vi "TestGridViewDotNET.vi"() -> ()   [LabVIEW 2013]
uses:
  Shared/LabVIEWdotNetDataGrid-master/source/GridColumn/ColumnDefinition.ctl
  Shared/LabVIEWdotNetDataGrid-master/source/GridColumn/ColumnType.ctl
  System.Windows.Forms
  Shared/LabVIEWdotNetDataGrid-master/source/DataGridView/DataGridView.lvclass
  Shared/LabVIEWdotNetDataGrid-master/source/Events/Abstract EVENT/Abstract EVENT.lvclass
  Shared/LabVIEWdotNetDataGrid-master/source/DataTable/DataTable.lvclass
  Shared/LabVIEWdotNetDataGrid-master/source/DataGridView/DataGridView.lvclass/DataGridView.ctl
  Shared/LabVIEWdotNetDataGrid-master/source/DataGridView/Properties/Read registeredEvents.vi
  Shared/LabVIEWdotNetDataGrid-master/source/DataTable/Add Rows (String).vi
  Shared/LabVIEWdotNetDataGrid-master/source/Events/CellValueChanged/CellValueChanged.lvclass
  Shared/LabVIEWdotNetDataGrid-master/source/Events/KeyDown/KeyDown.lvclass
  Shared/LabVIEWdotNetDataGrid-master/source/Events/CellClick/CellClick.lvclass
  Shared/LabVIEWdotNetDataGrid-master/source/GridColumn/GridColumn.lvclass
panel:
  in  "index":i32
  out "Events":string
  out "error out":errorcluster
  out "registeredEvents":refnum<event-registration>
  out "DataGrid out":refnum<class "DataGridView.lvclass">
  in  "error in":errorcluster
  in  "DataGridView":refnum<k24>(container)
  in  "ColumnSetup":T1[](array[typedef])=[{"name"="DeviceTypes", "caption"="DeviceTypes", "datatype"=enum."combo", "Params"="", "AutoSizeMode"=16, "FillWeight"=100.0, "MinWidth"=50, "tooltip"="DeviceTypes"}, {"name"="Devices", "caption"="Devices", "datatype"=enum."combo", "Params"="", "AutoSizeMode"=1, "FillWeight"=100.0, "MinWidth"=50, "tooltip"="Devices"}, {"name"="Variables", "caption"="Variables", "datatype"=enum."combo", "Params"="", "AutoSizeMode"=1, "FillWeight"=100.0, "MinWidth"=50, "tooltip"="Variables"}] {"MinWidth" min=2 step=1; "AutoSizeMode" items=["None"=1, "ColumnHeader"=2, "AllCellsExceptHeader"=4, "AllCells"=6, "DisplayedCellsExceptHeader"=8, "DisplayedCells"=10, "Fill"=16]; "FillWeight" min=1 max=100}
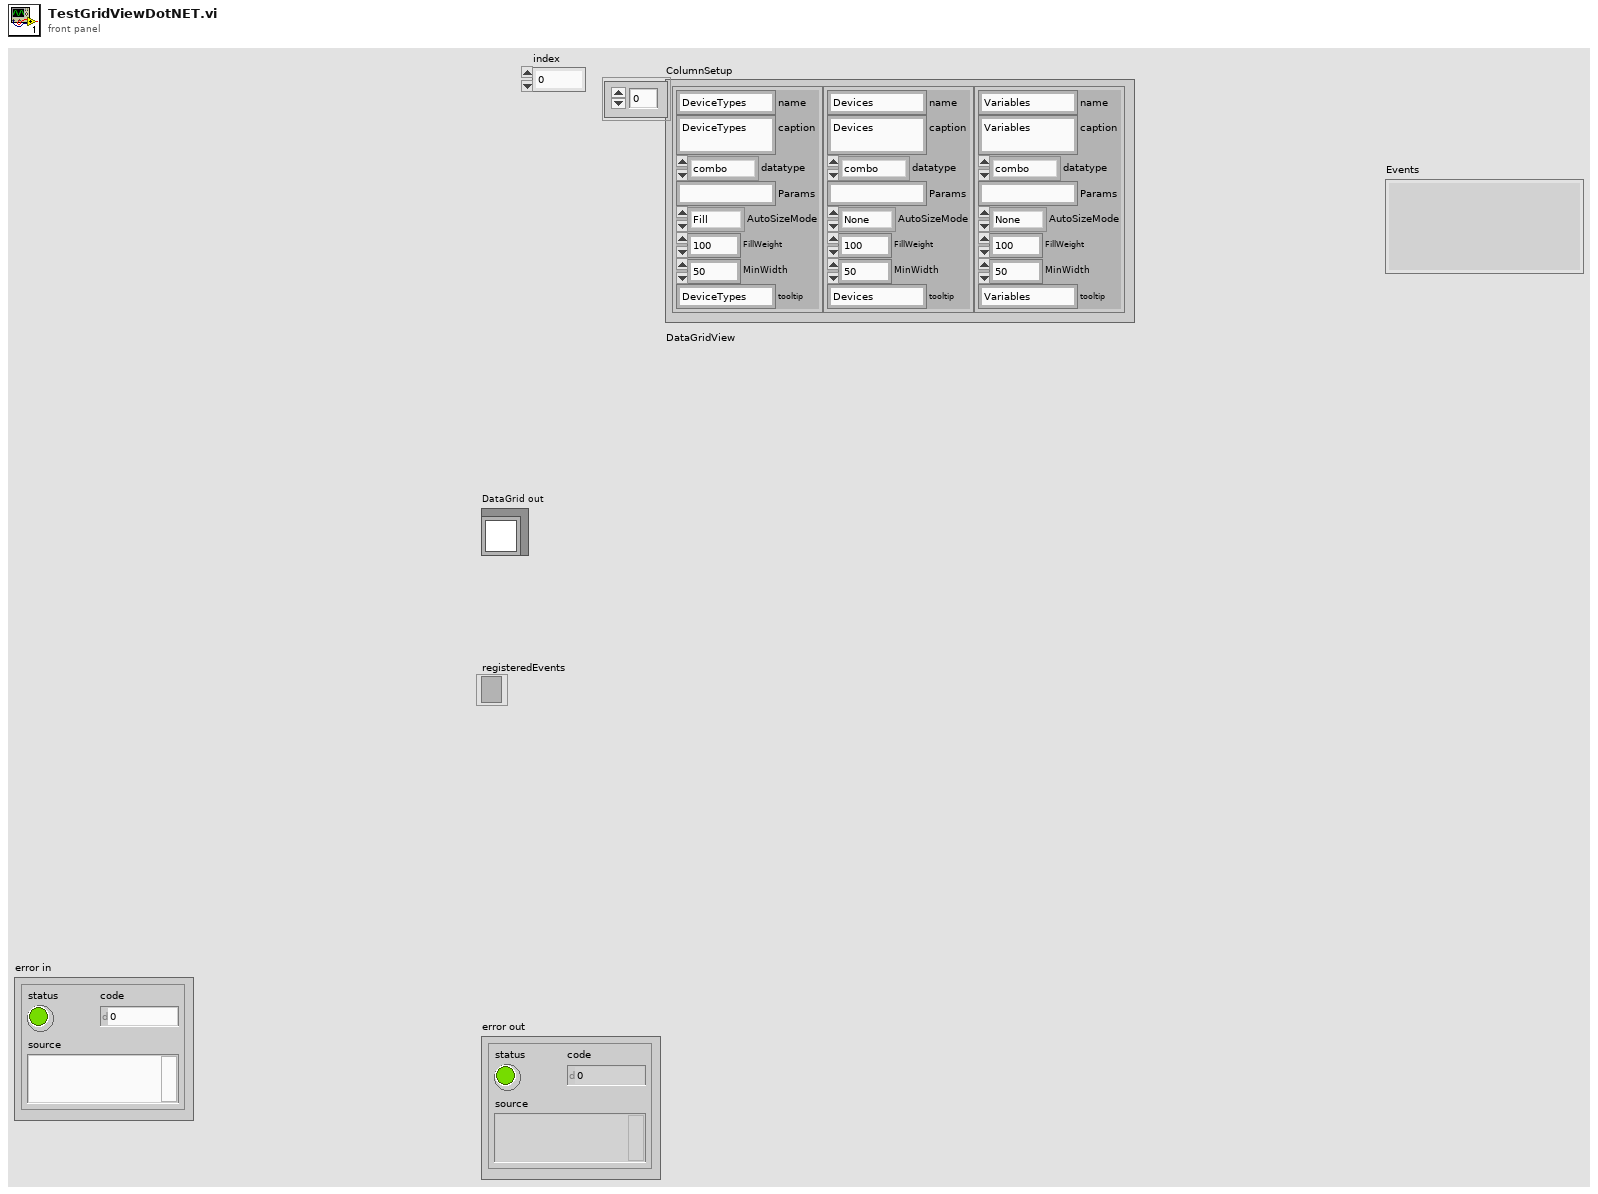
[diagram p1: front panel]
types:
  T1 = typedef "DataGrid.lvlib/GridColumn.lvclass/ColumnDefinition.ctl" = cluster{"name":string, "caption":string, "datatype":T2, "Params":string, "AutoSizeMode":i32, "FillWeight":sgl, "MinWidth":u32, "tooltip":string}
  T2 = typedef "DataGrid.lvlib/GridColumn.lvclass/ColumnType.ctl" = enum16{"string", "image", "check", "numeric", "timestamp", "button", "combo", "link"}
  T3 = cluster{"Alt":bool, "Control":bool, "KeyCode":i32, "KeyData":i32, "KeyValue":i32, "Modifiers":i32, "Shift":bool}
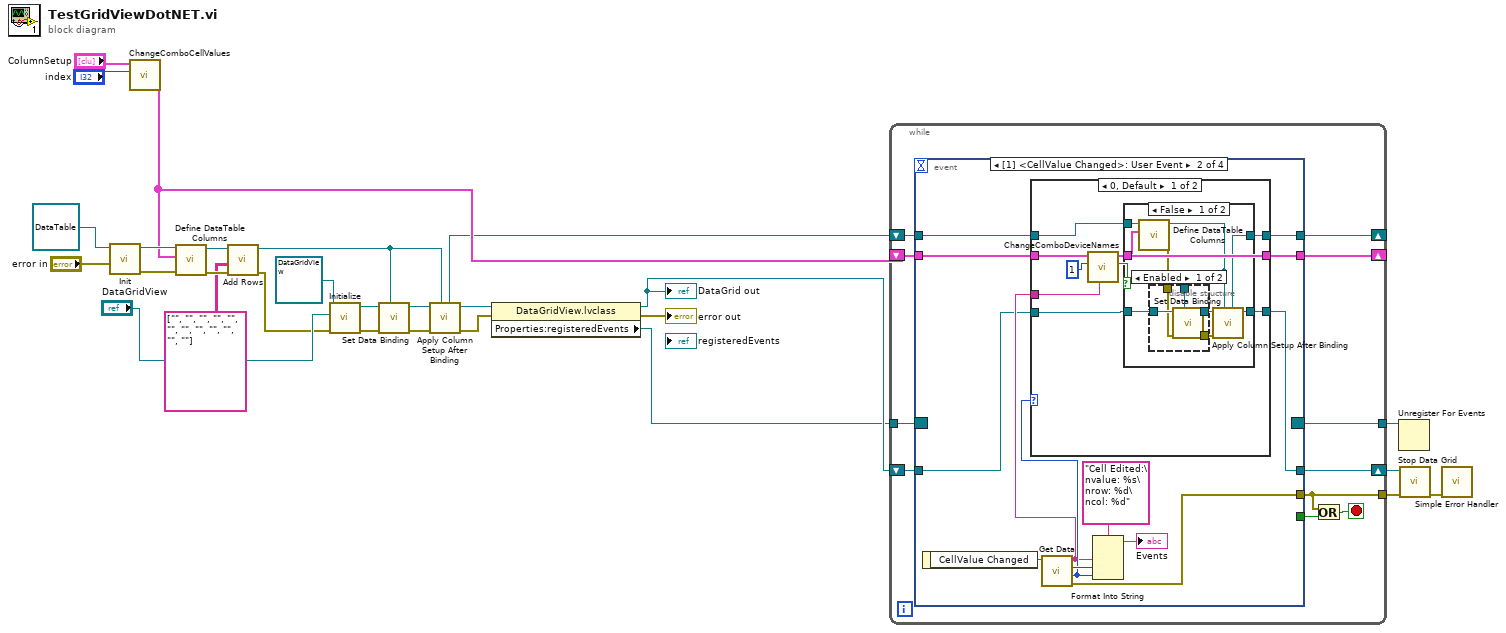
[diagram p0: block diagram]
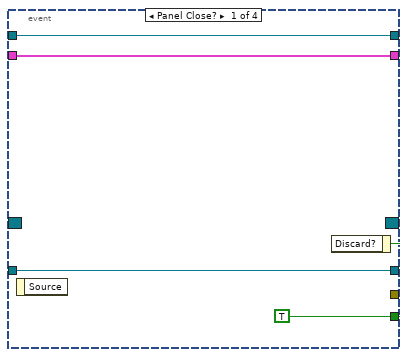
[diagram p2: hidden frame]
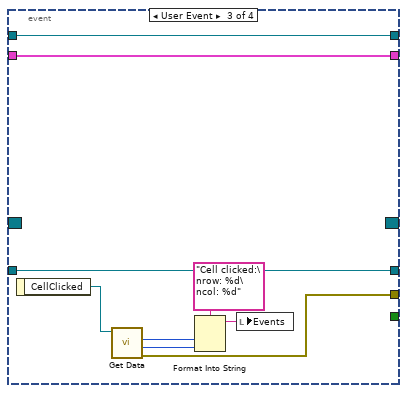
[diagram p6: hidden frame]
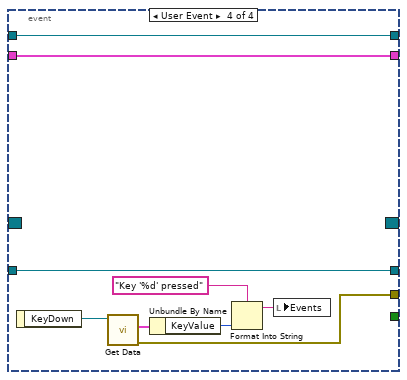
[diagram p7: hidden frame]
diagram:
  n1 = call "Init.vi"("error in (no error)"="error in", "DataTable in"=refnum<class "DataTable.lvclass"> refnum) -> ("error out"=w24:errorcluster, "DataTable out"=w25:refnum<class "DataTable.lvclass">)  [unwired: 8 in]
  n2 = call "ChangeComboCellValues.vi"("index"="index", "ColumnSetup in"="ColumnSetup") -> ("ColumnSetup out"=w5:T1[])  [unwired: 9 in]
  n3 = call "Define DataTable Columns.vi"("error in (no error)"=w24, "ColumnSetup"=w5, "DataTable In"=w25) -> ("error out"=w9:errorcluster, "DataTable Out"=w7:refnum<class "DataTable.lvclass">)  [unwired: 7 in]
  n4 = call-poly "Add Rows.vi"("error in (no error)"=w9, "String Data"=string[][] [["", "", ""], ["", "", ""], ["", "", ""], ["", "", ""]], "DataTable in"=w7) -> ("error out"=w8:errorcluster, "DataTable out"=w3:refnum<class "DataTable.lvclass">)  [unwired: 7 in]
  n5 = call "Initialize.vi"("error in"=w8, "DataGridView"="DataGridView", "DataGrid in"=refnum<class "DataGridView.lvclass"> refnum) -> ("error out"=w18:errorcluster, "DataGrid out"=w17:refnum<class "DataGridView.lvclass">)  [unwired: 7 in]
  n6 = call "Set Data Binding.vi"("DataTable Source"=w3, "error in (no error)"=w18, "DataGridView in"=w17) -> ("error out"=w21:errorcluster, "DataGridView out"=w23:refnum<class "DataGridView.lvclass">)  [unwired: 7 in]
  n7 = call "Apply Column Setup After Binding.vi"("DataTable"=w3, "error in (no error)"=w21, "DataGridView in"=w23) -> ("error out"=w19:errorcluster, "DataGridView out"=w22:refnum<class "DataGridView.lvclass">, "DataTable out"=w2:refnum<class "DataTable.lvclass">)  [unwired: 6 in]
  n8 = property class="DataGridView.lvclass"(reference=w22, error in=w19) -> (reference out=w10:refnum<class "DataGridView.lvclass">, error out=→"error out":errorcluster, "Properties:registeredEvents"=w1:refnum<event-registration>)
  "DataGrid out" <- w10
  n9 = while {
    tunnel: w1 -> [w39]
    shift-right: [w37] -> w12
    shift-left: w10 -> [w38]
    tunnel: [w36] -> w11
    tunnel: [w34] -> w13
    shift-right: [w31] -> _
    shift-left: w5 -> [w32]
    shift-right: [w29] -> _
    shift-left: w2 -> [w30]
    stop <- w33 stop-if-true
    n10 = event shown="[1] <CellValue Changed>: User Event" {
      selector: w39 -> [_ _ _ _]
      dyn-events: [_ _ _ _] -> w36
      timeout: _ -> [_ _ _ _]
      tunnel: [w43 _ _ _] -> w35
      tunnel: w38 -> [w42 w45 w94 w104]
      tunnel: [w42 w44 w94 w104] -> w37
      tunnel: [_ w52 w91 w98] -> w34
      tunnel: w32 -> [w41 w51 w88 w97]
      tunnel: [w41 w48 w88 w97] -> w31
      tunnel: w30 -> [w40 w47 w87 w96]
      tunnel: [w40 w46 w87 w96] -> w29
      event Panel Close? {
        w43 = TRUE ("Discard?")
        n11 = event-data() -> ()  [unwired: 1 in, 1 out]
        n12 = event-data("Discard?"=w43) -> ()  [unwired: 1 in, 1 out]
      }
      event User Event {
        n13 = event-data() -> ("CellValue Changed"=w54:refnum<class "Abstract EVENT.lvclass">)  [unwired: 1 in]
        n14 = call "Get Data.vi"("DataGrid.lvlib:Abstract EVENT.lvclass"=w54) -> ("error out"=w52:errorcluster, "column"=w50:i32, "row"=w53:i32, "cell value"=w49:string)  [unwired: 7 in]
        n15 = case shown="0, Default" w50 {
          tunnel: w51 -> [w65 w86]
          tunnel: w49 -> [w63 _]
          tunnel: [w58 w86] -> w48
          tunnel: w47 -> [w60 w85]
          tunnel: [w59 w85] -> w46
          tunnel: w45 -> [w61 w84]
          tunnel: [w62 w84] -> w44
          frame 0, Default {
            n16 = call "ChangeComboDeviceNames.vi"("DeviceTypeName"=w63, "index"=1, "ColumnSetup in"=w65) -> ("empty?"=w57:bool, "ColumnSetup out"=w58:T1[])  [unwired: 7 in]
            n17 = case shown="False" w57 {
              tunnel: [w74 w82] -> w62
              tunnel: w61 -> [w72 w82]
              tunnel: w60 -> [w70 w83]
              tunnel: [w66 w83] -> w59
              tunnel: w58 -> [w67 _]
              frame False {
                n18 = call "Define DataTable Columns.vi"("ColumnSetup"=w67, "DataTable In"=w70) -> ("error out"=w68:errorcluster, "DataTable Out"=w69:refnum<class "DataTable.lvclass">)  [unwired: 8 in]
                n19 = disable-structure shown="Enabled" {
                  disable-tunnel: [w79 w80] -> w73
                  disable-tunnel: w72 -> [w78 w81]
                  disable-tunnel: [w77 w81] -> w71
                  disable-tunnel: w69 -> [w76 _]
                  disable-tunnel: w68 -> [w75 w80]
                  frame Enabled {
                    n20 = call "Set Data Binding.vi"("DataTable Source"=w76, "error in (no error)"=w75, "DataGridView in"=w78) -> ("error out"=w79:errorcluster, "DataGridView out"=w77:refnum<class "DataGridView.lvclass">)  [unwired: 7 in]
                  }
                  frame Disabled {
                  }
                }
                n21 = call "Apply Column Setup After Binding.vi"("DataTable"=w69, "error in (no error)"=w73, "DataGridView in"=w71) -> ("DataGridView out"=w74:refnum<class "DataGridView.lvclass">, "DataTable out"=w66:refnum<class "DataTable.lvclass">)  [unwired: 6 in, 1 out]
              }
              frame True {
              }
            }
          }
          frame 1 {
          }
        }
        n22 = Format Into String(format string="Cell Edited:\nvalue: %s\nrow: %d\ncol: %d" ("message"), w49, w53, w50) -> (resulting string=→"Events":string)  [unwired: 2 in, 1 out]
      }
      event User Event {
        n23 = event-data() -> ("CellClicked"=w92:refnum<class "Abstract EVENT.lvclass">)  [unwired: 1 in]
        n24 = call "Get Data.vi"("DataGrid.lvlib:Abstract EVENT.lvclass"=w92) -> ("error out"=w91:errorcluster, "column"=w90:i32, "row"=w89:i32)  [unwired: 8 in]
        n25 = Format Into String(format string="Cell clicked:\nrow: %d\ncol: %d" ("message"), w89, w90) -> (resulting string=w95:string)  [unwired: 2 in, 1 out]
        n26 = local write "Events"(w95) -> ()
      }
      event User Event {
        n27 = event-data() -> ("KeyDown"=w103:refnum<class "Abstract EVENT.lvclass">)  [unwired: 1 in]
        n28 = call "Get Data.vi"("DataGrid.lvlib:Abstract EVENT.lvclass"=w103) -> ("error out"=w98:errorcluster, "output cluster"=w100:T3)  [unwired: 9 in]
        n29 = Unbundle By Name(w100) -> ("KeyValue"=w99:i32)
        n30 = Format Into String(format string="Key '%d' pressed" ("message"), w99) -> (resulting string=w102:string)  [unwired: 2 in, 1 out]
        n31 = local write "Events"(w102) -> ()
      }
    }
    n32 = Or(x=w34, y=w35) -> (x .or. y?=w33:bool)
  }
  n33 = Unregister For Events(event registration refnum=w11) -> ()  [unwired: 1 in, 1 out]
  n34 = call "Stop Data Grid.vi"("error in (no error)"=w13, "DataGridView in"=w12) -> ("error out"=w14:errorcluster)  [unwired: 8 in, 1 out]
  n35 = call <vilib>:"Simple Error Handler.vi"("error in (no error)"=w14) -> ()  [unwired: 4 in, 5 out]
